vi "Read Post Offices.vi"(8 "error in (no error)":errorcluster, 11 "Factory in":refnum<class "Factory.lvclass">) -> (0 "error out":errorcluster, 3 "Factory out":refnum<class "Factory.lvclass">)   [LabVIEW 2019, in "Factory.lvclass"]
uses:
  Factory.lvclass
  Factory.lvclass/Factory.ctl
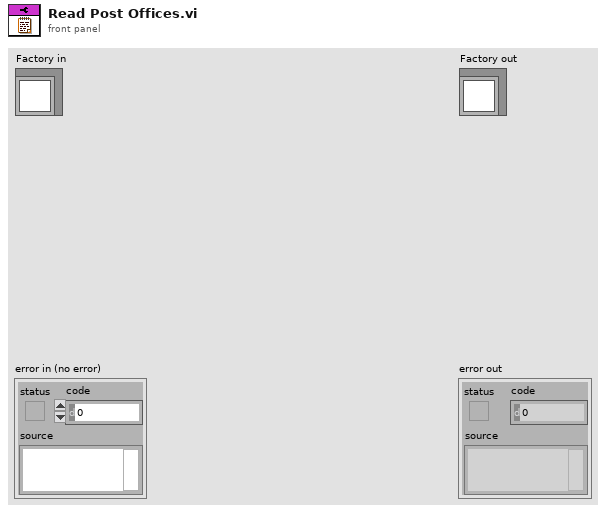
[diagram p1: front panel]
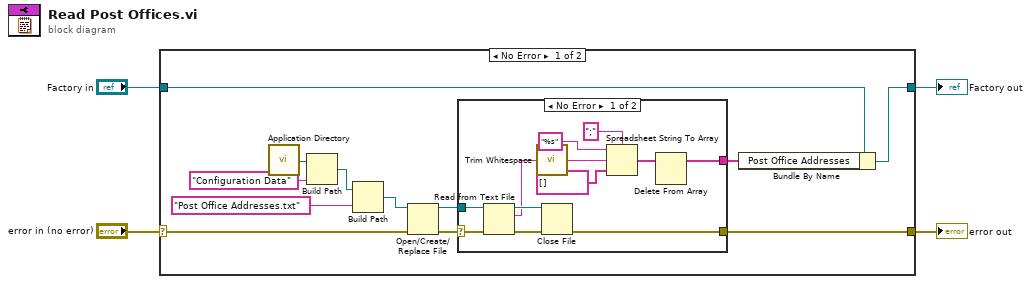
[diagram p0: block diagram]
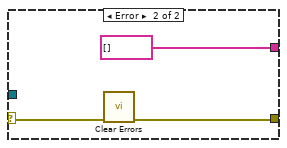
[diagram p2: hidden frame]
diagram:
  n1 = case shown="No Error" "error in (no error)" {
    selector: "error in (no error)" -> [w12 w33]
    tunnel: [w8 w33] -> w3
    tunnel: [w5 w32] -> w1
    tunnel: "Factory in" -> [w7 w32]
    frame No Error {
      n2 = call <vilib>:"Application Directory.vi"() -> ("Application Directory"=w16:path)
      n3 = Build Path(base path=w16, name or relative path="Configuration Data") -> (appended path=w14:path)
      n4 = Build Path(base path=w14, name or relative path="Post Office Addresses.txt") -> (appended path=w11:path)
      n5 = Open/Create/Replace File(file path (use dialog)=w11, error in=w12) -> (refnum out=w9:refnum<file>, error out=w10:errorcluster)  [unwired: 4 in, 1 out]
      n6 = case shown="No Error" w10 {
        selector: w10 -> [w28 w31]
        tunnel: w9 -> [w27 _]
        tunnel: [w17 string[] [] ("delimiter (Tab)")] -> w6
        tunnel: [w19 w30] -> w8
        frame No Error {
          n7 = Read from Text File(file (use dialog)=w27, error in=w28) -> (refnum out=w25:refnum<file>, text=w24:string, error out=w26:errorcluster)  [unwired: 2 in, 1 out]
          n8 = call <vilib>:"Trim Whitespace.vi"("string"=w24) -> ("trimmed string"=w22:string)  [unwired: 1 in]
          n9 = Close File(refnum=w25, error in=w26) -> (error out=w19:errorcluster)  [unwired: 1 out]
          n10 = Spreadsheet String To Array(delimiter (Tab)=";", format string="%s", spreadsheet string=w22, array type (2D Dbl)=string[] [] ("delimiter (Tab)")) -> (array=w18:string[])
          n11 = Delete From Array(array=w18) -> (array with subset deleted=w17:string[])  [unwired: 2 in, 1 out]
        }
        frame Error {
          n12 = call <vilib>:"Clear Errors.vi"("error in (no error)"=w31) -> ("error out"=w30:errorcluster)  [unwired: 5 in, 1 out]
        }
      }
      n13 = Bundle By Name(cluster=w7, "Post Office Addresses"=w6) -> (w5:refnum<class "Factory.lvclass">)
    }
    frame Error {
    }
  }
  "error out" <- w3
  "Factory out" <- w1
